vi "populateTrajectory.vi"(6 "ptDuration (ms)":i32=20, 7 "loopTime (ms)":u32, 8 "rightDriveTraj":dbl[][](array[numeric]), 9 "rightDrive":T1={"DeviceStatus"={"status"=FALSE, "code"=0, "source"=""}, "Type"=enum."PWM", "PWM"={"PWM Channel"=enum."Invalid", "DeadBand"={"Name"="", "maxPositivePwm"=0, "minPositivePwm"=0, "centerPwm"=0, "maxNegativePwm"=0, "minNegativePwm"=0, "angularRange"=0}}, "CAN"={"Device Number"=0, "SetOutput VI Ref"=variant, "GetOutput VI Ref"=variant, "Enable VI Ref"=variant, "Disable VI Ref"=variant, "Data"=variant}, "Invert"=FALSE, "DIO PWM"={"PWM \"Enable\" Channel"=enum."Invalid", "DIOChannel"=enum."Invalid", "PWM Rate"=0.0}}, 10 "leftDriveTraj":dbl[][](array[numeric]), 11 "leftDrive":T1={"DeviceStatus"={"status"=FALSE, "code"=0, "source"=""}, "Type"=enum."PWM", "PWM"={"PWM Channel"=enum."Invalid", "DeadBand"={"Name"="", "maxPositivePwm"=0, "minPositivePwm"=0, "centerPwm"=0, "maxNegativePwm"=0, "minNegativePwm"=0, "angularRange"=0}}, "CAN"={"Device Number"=0, "SetOutput VI Ref"=variant, "GetOutput VI Ref"=variant, "Enable VI Ref"=variant, "Disable VI Ref"=variant, "Data"=variant}, "Invert"=FALSE, "DIO PWM"={"PWM \"Enable\" Channel"=enum."Invalid", "DIOChannel"=enum."Invalid", "PWM Rate"=0.0}}) -> ()   [LabVIEW 2017]
uses:
  <vilib>/Rock Robotics/WPI/MotorControl/WPI_MotorControlDeviceRef.ctl
  <vilib>/Rock Robotics/WPI/MotorControl/WPI_MotorControlType.ctl
  <vilib>/Rock Robotics/SystemInterfaces/DIO/FPGA_DIOPWMChannel.ctl
  <vilib>/Rock Robotics/WPI/PWM/WPI_PWMDeadband.ctl
  <vilib>/Rock Robotics/SystemInterfaces/DIO/FPGA_DIOChannel.ctl
  <vilib>/Rock Robotics/WPI/ThirdParty/Phoenix-LabVIEW/Motor Controller/Controls/CTRE_Phoenix_MotorControl_TrajectoryPointTimeDur.ctl
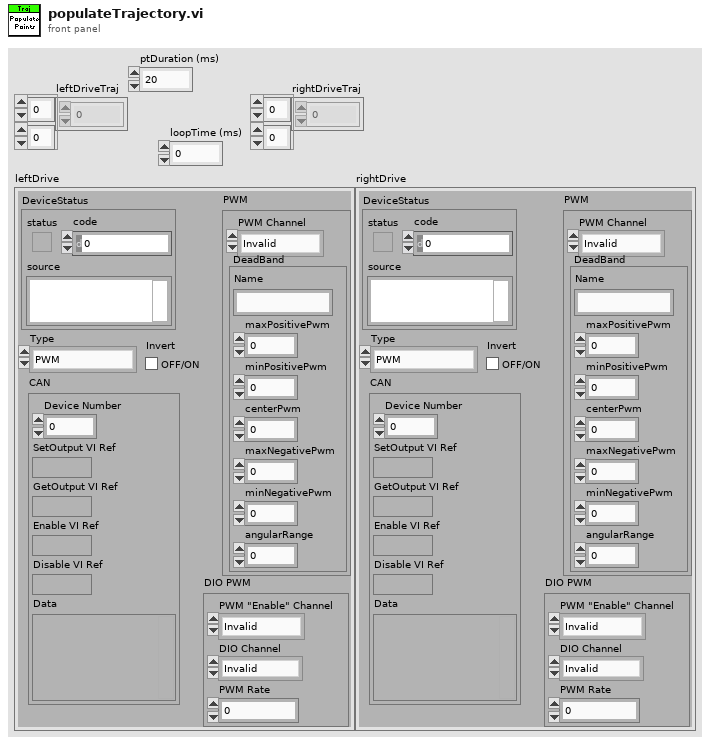
[diagram p1: front panel]
types:
  T1 = typedef "WPI_MotorControlDeviceRef.ctl" = cluster{"DeviceStatus":errorcluster, "Type":T2, "PWM":cluster{"PWM Channel":T3, "DeadBand":T4}, "CAN":cluster{"Device Number":u8, "SetOutput VI Ref":variant, "GetOutput VI Ref":variant, "Enable VI Ref":variant, "Disable VI Ref":variant, "Data":variant}, "Invert":bool, "DIO PWM":cluster{"PWM \"Enable\" Channel":T3, "DIOChannel":T5, "PWM Rate":dbl}}
  T2 = typedef "WPI_MotorControlType.ctl" = enum16{"PWM", "CAN", "DIO PWM"}
  T3 = typedef "FPGA_DIOPWMChannel.ctl" = enum8{"PWM 0", "PWM 1", "PWM 2", "PWM 3", "PWM 4", "PWM 5", "PWM 6", "PWM 7", "PWM 8", "PWM 9", "PWM MXP 0", "PWM MXP 1", "PWM MXP 2", "PWM MXP 3", "PWM MXP 4", "PWM MXP 5", "PWM MXP 6", "PWM MXP 7", "PWM MXP 8", "PWM MXP 9", "Invalid"}
  T4 = typedef "WPI_PWMDeadband.ctl" = cluster{"Name":string, "maxPositivePwm":i32, "minPositivePwm":i32, "centerPwm":i32, "maxNegativePwm":i32, "minNegativePwm":i32, "angularRange":u16}
  T5 = typedef "FPGA_DIOChannel.ctl" = enum8{"DIO 0", "DIO 1", "DIO 2", "DIO 3", "DIO 4", "DIO 5", "DIO 6", "DIO 7", "DIO 8", "DIO 9", "DIO MXP 0", "DIO MXP 1", "DIO MXP 2", "DIO MXP 3", "DIO MXP 4", "DIO MXP 5", "DIO MXP 6", "DIO MXP 7", "DIO MXP 8", "DIO MXP 9", "DIO MXP 10", "DIO MXP 11", "DIO MXP 12", "DIO MXP 13", "DIO MXP 14", "DIO MXP 15", "SPI Port CS1", "SPI Port CS2", "SPI Port CS3", "SPI Port MISO", "SPI Port MOSI", "Invalid"}
  T6 = typedef "CTRE_Phoenix_MotorControl_TrajectoryPointTimeDur.ctl" = i32
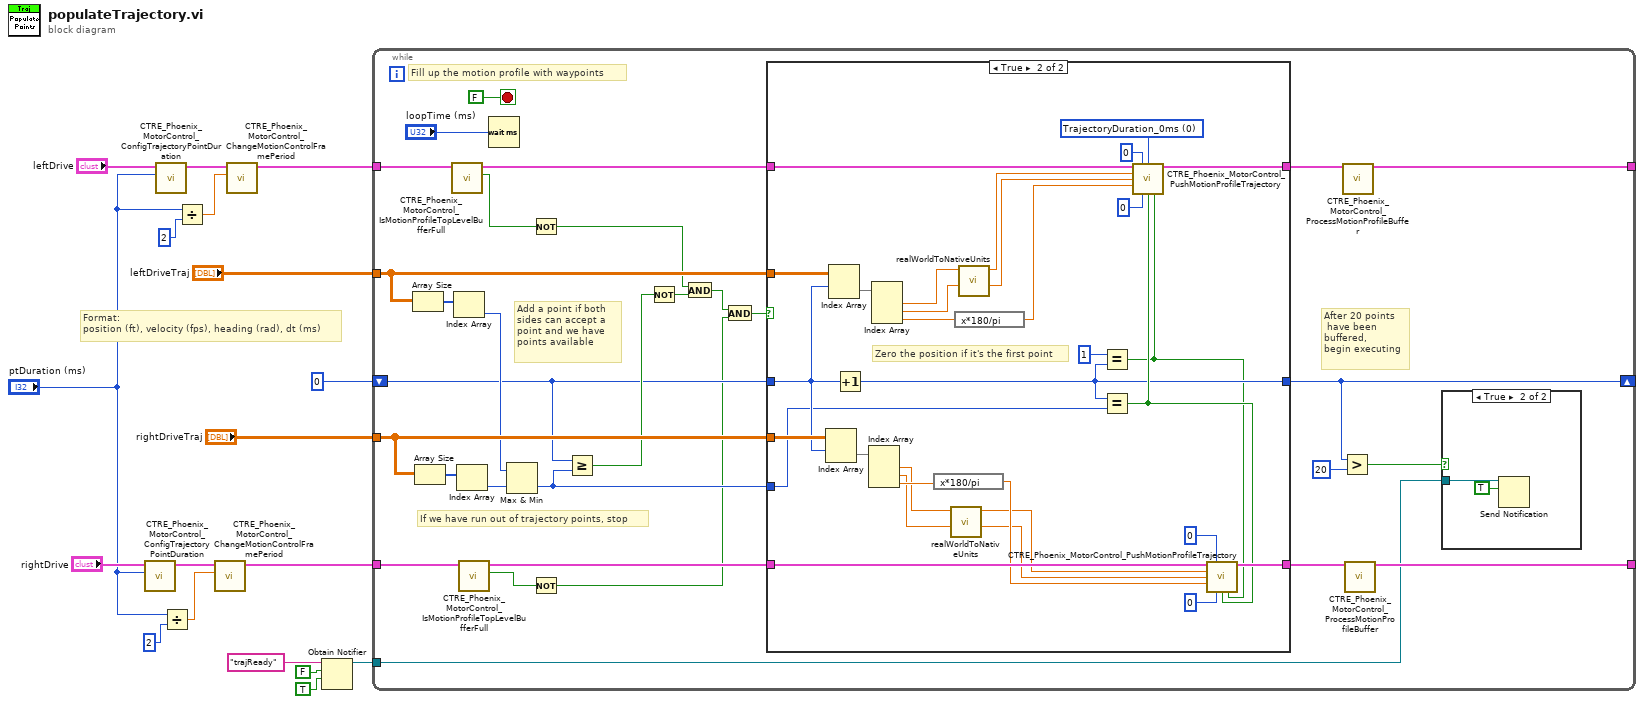
[diagram p0: block diagram]
diagram:
  # "Format:\nposition (ft), velocity (fps), heading (rad), dt (ms)"
  n1 = call <vilib>:"CTRE_Phoenix_MotorControl_ConfigTrajectoryPointDuration.vi"("durationMs"="ptDuration (ms)", "PhoenixMotorControlDevRef"="rightDrive") -> ("PhoenixMotorControlDevRef"=w15:T1)  [unwired: 8 in, 1 out]
  n2 = call <vilib>:"CTRE_Phoenix_MotorControl_ConfigTrajectoryPointDuration.vi"("durationMs"="ptDuration (ms)", "PhoenixMotorControlDevRef"="leftDrive") -> ("PhoenixMotorControlDevRef"=w12:T1)  [unwired: 8 in, 1 out]
  n3 = Divide(x="ptDuration (ms)", y=2) -> (x/y=w8:dbl)
  n4 = Divide(x="ptDuration (ms)", y=2) -> (x/y=w11:dbl)
  n5 = call <vilib>:"CTRE_Phoenix_MotorControl_ChangeMotionControlFramePeriod.vi"("periodMs"=w8, "PhoenixMotorControlDevRef"=w15) -> ("PhoenixMotorControlDevRef"=w14:T1)  [unwired: 8 in, 1 out]
  n6 = call <vilib>:"CTRE_Phoenix_MotorControl_ChangeMotionControlFramePeriod.vi"("periodMs"=w11, "PhoenixMotorControlDevRef"=w12) -> ("PhoenixMotorControlDevRef"=w13:T1)  [unwired: 8 in, 1 out]
  n7 = Obtain Notifier(name (unnamed)="trajReady", notification data type=FALSE, create if not found? (T)=TRUE) -> (notifier out=w2:refnum<notifier>)  [unwired: 1 in, 2 out]
  n8 = while {
    shift-right: [w22] -> _
    shift-left: 0 -> [w38]
    tunnel: "leftDriveTraj" -> [w48]
    tunnel: "rightDriveTraj" -> [w47]
    tunnel: w13 -> [w32]
    tunnel: w14 -> [w36]
    tunnel: [w24] -> _
    tunnel: [w23] -> _
    tunnel: w2 -> [w19]
    stop <- FALSE stop-if-true
    # "After 20 points\n have been\nbuffered, \nbegin executing"
    # "Add a point if both \nsides can accept a\npoint and we have\npoints available"
    # "If we have run out of trajectory points, stop"
    # "Fill up the motion profile with waypoints"
    n9 = Array Size(array=w48) -> (size(s)=w44:i32[])
    n10 = Array Size(array=w47) -> (size(s)=w45:i32[])
    n11 = call <vilib>:"CTRE_Phoenix_MotorControl_IsMotionProfileTopLevelBufferFull.vi"("PhoenixMotorControlDevRef"=w32) -> ("Is Motion Profile Top Level Buffer Full?"=w30:bool, "PhoenixMotorControlDevRef"=w31:T1)  [unwired: 8 in, 1 out]
    n12 = Index Array(array=w44) -> (element=w43:i32)  [unwired: 1 in]
    n13 = Index Array(array=w45) -> (element=w46:i32)  [unwired: 1 in]
    n14 = call <vilib>:"CTRE_Phoenix_MotorControl_IsMotionProfileTopLevelBufferFull.vi"("PhoenixMotorControlDevRef"=w36) -> ("Is Motion Profile Top Level Buffer Full?"=w34:bool, "PhoenixMotorControlDevRef"=w35:T1)  [unwired: 8 in, 1 out]
    n15 = Wait (ms)(milliseconds to wait="loopTime (ms)") -> ()  [unwired: 1 out]
    n16 = Max & Min(x=w43, y=w46) -> (min(x,y)=w37:i32)  [unwired: 1 out]
    n17 = Not(x=w30) -> (.not. x?=w29:bool)
    n18 = Not(x=w34) -> (.not. x?=w33:bool)
    n19 = Greater Or Equal?(x=w38, y=w37) -> (x >= y?=w39:bool)
    n20 = Not(x=w39) -> (.not. x?=w40:bool)
    n21 = And(x=w29, y=w40) -> (x .and. y?=w41:bool)
    n22 = And(x=w41, y=w33) -> (x .and. y?=w42:bool)
    n23 = case shown="True" w42 {
      tunnel: w38 -> [w53 w80]
      tunnel: [w53 w57] -> w22
      tunnel: w48 -> [_ w83]
      tunnel: w47 -> [_ w81]
      tunnel: w31 -> [w51 w77]
      tunnel: w35 -> [w52 w79]
      tunnel: [w52 w78] -> w27
      tunnel: [w51 w76] -> w28
      tunnel: w37 -> [_ w60]
      frame False {
      }
      frame True {
        w54 = T6 0 items=["TrajectoryDuration_0ms"=0, "TrajectoryDuration_5ms"=5, "TrajectoryDuration_10ms"=10, "TrajectoryDuration_20ms"=20, "TrajectoryDuration_30ms"=30, "TrajectoryDuration_40ms"=40, "TrajectoryDuration_50ms"=50, "TrajectoryDuration_100ms"=100] ("durationMs")
        # "Zero the position if it's the first point"
        n24 = Index Array(array=w81, index (row)=w80) -> (element=w82:dbl[])  [unwired: 1 in]
        n25 = Index Array(array=w83, index (row)=w80) -> (element=w84:dbl[])  [unwired: 1 in]
        n26 = Increment(x=w80) -> (x+1=w57:i32)
        n27 = Index Array(array=w82) -> (element #1=w68:dbl, element #2=w69:dbl, element #3=w71:dbl)  [unwired: 3 in]
        n28 = Index Array(array=w84) -> (element #1=w66:dbl, element #2=w67:dbl, element #3=w73:dbl)  [unwired: 3 in]
        n29 = expression code="x*180/pi"(w71) -> (w70:dbl)
        n30 = call "realWorldToNativeUnits.vi"("velocity (ft/s)"=w69, "position (ft)"=w68) -> ("velocity (u/100ms)"=w62:dbl, "position (u)"=w63:dbl)  [unwired: 8 in]
        n31 = expression code="x*180/pi"(w73) -> (w72:dbl)
        n32 = call "realWorldToNativeUnits.vi"("velocity (ft/s)"=w67, "position (ft)"=w66) -> ("velocity (u/100ms)"=w64:dbl, "position (u)"=w65:dbl)  [unwired: 8 in]
        n33 = Equal?(x=1, y=w57) -> (x = y?=w55:bool)
        n34 = Equal?(x=w57, y=w60) -> (x = y?=w61:bool)
        n35 = call <vilib>:"CTRE_Phoenix_MotorControl_PushMotionProfileTrajectory.vi"("PhoenixMotorControlDevRef"=w77, "profileSlotSelect1"=0, "durationMs"=w54, "position"=w65, "velocity"=w64, "auxiliaryPos"=w72, "profileSlotSelect0"=0, "isLastPoint?"=w61, "Zero Position?"=w55) -> ("PhoenixMotorControlDevRef"=w76:T1)  [unwired: 5 in, 1 out]
        n36 = call <vilib>:"CTRE_Phoenix_MotorControl_PushMotionProfileTrajectory.vi"("PhoenixMotorControlDevRef"=w79, "profileSlotSelect1"=0, "position"=w63, "velocity"=w62, "auxiliaryPos"=w70, "profileSlotSelect0"=0, "isLastPoint?"=w61, "Zero Position?"=w55) -> ("PhoenixMotorControlDevRef"=w78:T1)  [unwired: 6 in, 1 out]
      }
    }
    n37 = Greater?(x=w22, y=20) -> (0:w20:bool)
    n38 = call <vilib>:"CTRE_Phoenix_MotorControl_ProcessMotionProfileBuffer.vi"("PhoenixMotorControlDevRef"=w28) -> ("PhoenixMotorControlDevRef"=w24:T1)  [unwired: 13 in, 1 out]
    n39 = call <vilib>:"CTRE_Phoenix_MotorControl_ProcessMotionProfileBuffer.vi"("PhoenixMotorControlDevRef"=w27) -> ("PhoenixMotorControlDevRef"=w23:T1)  [unwired: 13 in, 1 out]
    n40 = case shown="True" w20 {
      tunnel: w19 -> [_ w50]
      frame False {
      }
      frame True {
        n41 = Send Notification(notification=TRUE, notifier=w50) -> ()  [unwired: 1 in, 2 out]
      }
    }
  }
